vi "Constrain Object into Pane.vi"(4 "Pane Bounds":T1, 6 "Panel Origin":T2, 8 "Error In":errorcluster, 10 "Object Size":T1, 11 "Object Position in":T3) -> (0 "Error Out":errorcluster, 3 "Object Position out":T3)   [LabVIEW 2019]
uses:
  <vilib>/Utility/miscctls.llb/LVPositionTypeDef.ctl
  <vilib>/Utility/miscctls.llb/LVBoundsTypeDef.ctl
  <vilib>/Utility/miscctls.llb/LVPointTypeDef.ctl
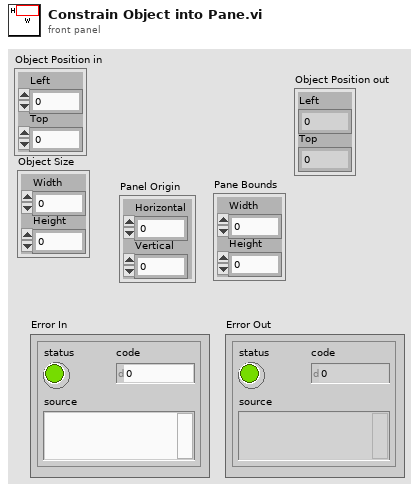
[diagram p1: front panel]
types:
  T1 = typedef "LVBoundsTypeDef.ctl" = cluster{"Width":u32, "Height":u32}
  T2 = typedef "LVPointTypeDef.ctl" = cluster{"Horizontal":i16, "Vertical":i16}
  T3 = typedef "LVPositionTypeDef.ctl" = cluster{"Left":i32, "Top":i32}
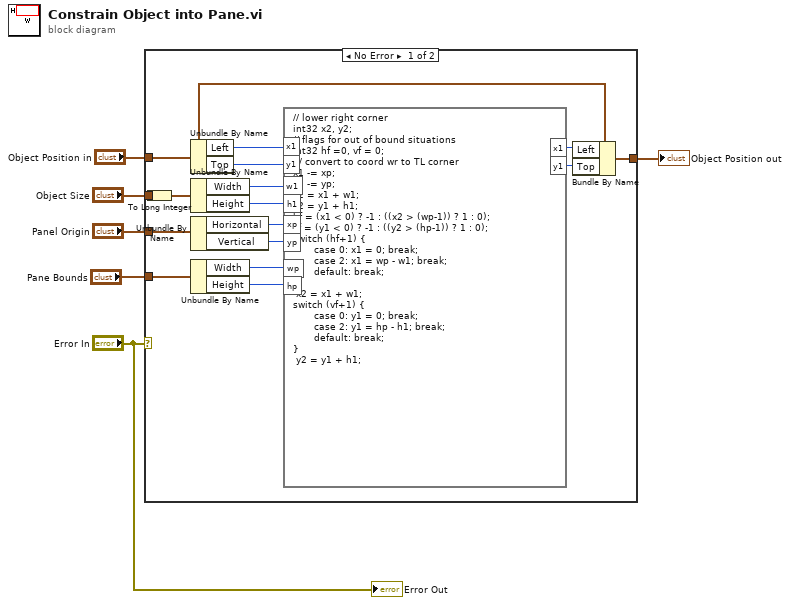
[diagram p0: block diagram]
diagram:
  n1 = case shown="No Error" "Error In" {
    tunnel: "Object Size" -> [w22 _]
    tunnel: "Panel Origin" -> [w16 _]
    tunnel: "Pane Bounds" -> [w13 _]
    tunnel: "Object Position in" -> [w10 w23]
    tunnel: [w7 w23] -> w2
    frame No Error {
      n2 = To Long Integer(number=w22) -> (32bit integer=w19:cluster{"Width":i32, "Height":i32})
      n3 = Unbundle By Name(w10) -> ("Left"=w21:i32, "Top"=w20:i32)
      n4 = Unbundle By Name(w19) -> ("Width"=w18:i32, "Height"=w17:i32)
      n5 = Unbundle By Name(w16) -> ("Horizontal"=w15:i16, "Vertical"=w14:i16)
      n6 = Unbundle By Name(w13) -> ("Width"=w12:u32, "Height"=w11:u32)
      n7 = formula code="// lower right corner\nint32 x2, y2;\n// flags for out of bound situations\nint32 hf =0, vf = 0;\n // convert to coord wr to TL corner\nx1 -= xp;\ny1 -= yp;\nx2 = x1 + w1;\ny2 = y1 + h1;\nhf = (x1 < 0) ? -1 : ((x2 > (wp-1)) ? 1 : 0);\nvf = (y1 < 0) ? -1 : ((y2 > (hp-1)) ? 1 : 0);\nswitch (hf+1) {\n       case 0: x1 = 0; break;\n       case 2: x1 = wp - w1; break;\n       default: break;\n}\n x2 = x1 + w1; \nswitch (vf+1) {\n       case 0: y1 = 0; break;\n       case 2: y1 = hp - h1; break;\n       default: break;\n}\n y2 = y1 + h1;"("x1"=w21, "y1"=w20, "w1"=w18, "h1"=w17, "xp"=w15, "yp"=w14, "wp"=w12, "hp"=w11) -> ("x1"=w9:i32, "y1"=w8:i32)
      n8 = Bundle By Name(cluster=w10, "Left"=w9, "Top"=w8) -> (w7:T3)
    }
    frame Error {
    }
  }
  "Object Position out" <- w2
  "Error Out" <- "Error In"
